vi "BuildWindow.vi"(8 "error in (no error)":errorcluster, 11 "AnalysisPluginsBase in":refnum<class "AnalysisPluginsBase.lvclass">) -> (0 "error out":errorcluster, 3 "AnalysisPluginsBase out":refnum<class "AnalysisPluginsBase.lvclass">)   [LabVIEW 2014]
uses:
  AnalysisPluginsBase.lvclass
  Typedefs/clWindowData.ctl
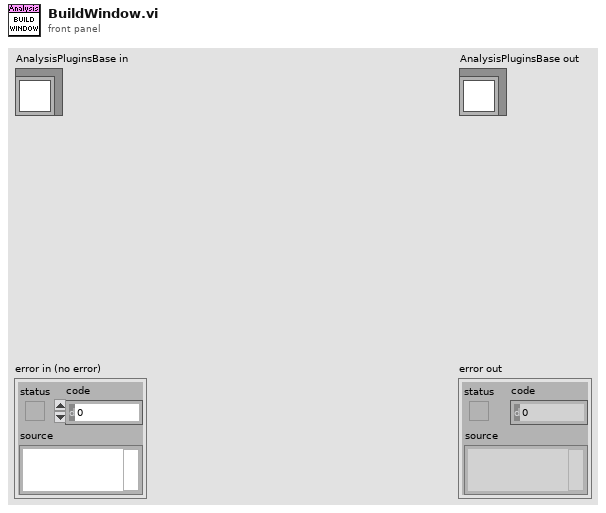
[diagram p1: front panel]
types:
  T1 = typedef "clWindowData.ctl" = cluster{"Timestamp":ext, "Samples":dbl[][], "Window Valid":bool}
  T2 = typedef "AnalysisPlugins.lvlib/AnalysisPluginsBase.lvclass/SampleDataInput.ctl" = T3[]
  T3 = typedef "AnalysisPlugins.lvlib/AnalysisPluginsBase.lvclass/clSampleData.ctl" = cluster{"Timestamp":ext, "SampleDataInput":cluster{"dSampleData":dbl[], "iActualPts":i32}[]}
  T4 = typedef "AnalysisPlugins.lvlib/AnalysisPluginsBase.lvclass/clConfig.ctl" = cluster{"F0":u32, "SettlingTime":dbl, "AnalysisCycles":dbl, "SampleRate":dbl, "NumChannels":u32, "TsOffset":enum16{"start", "middle", "end"}}
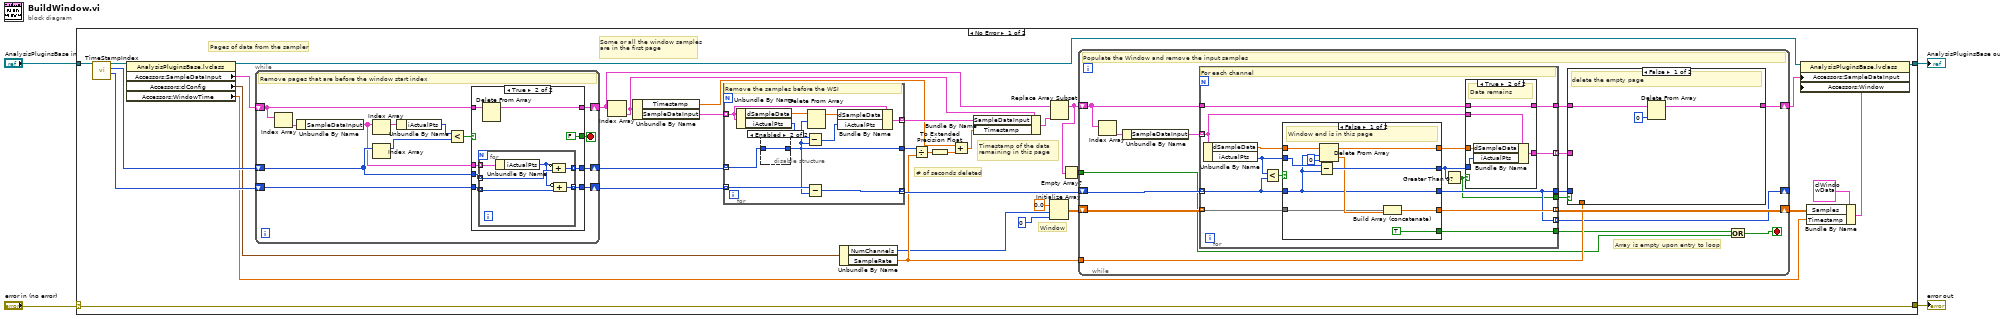
[diagram p0: block diagram]
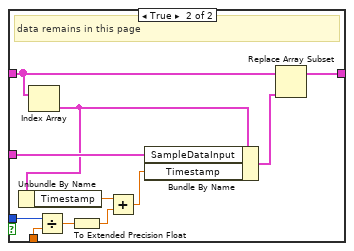
[diagram p2: hidden frame]
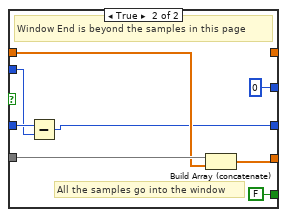
[diagram p4: hidden frame]
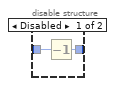
[diagram p5: hidden frame]
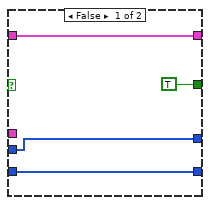
[diagram p6: hidden frame]
diagram:
  n1 = case shown="No Error" "error in (no error)" {
    selector: "error in (no error)" -> [w38 w153]
    tunnel: [w38 w153] -> w3
    tunnel: [w20 w152] -> w1
    tunnel: "AnalysisPluginsBase in" -> [w37 w152]
    frame No Error {
      # "Window"
      # "Timestamp of the data remaining in this page"
      # "# of seconds deleted"
      # "Pages of data from the sampler"
      # "Some or all the window samples are in the first page"
      n2 = call "TimeStampIndex.vi"("Analysis In"=w37) -> ("WEI"=w33:i32[], "WSI"=w34:i32[], "Analysis Out"=w36:refnum<class "AnalysisPluginsBase.lvclass">)  [unwired: 8 in]
      n3 = property class="AnalysisPluginsBase.lvclass"(reference=w36) -> (reference out=w21:refnum<class "AnalysisPluginsBase.lvclass">, "Accessors:SampleDataInput"=w35:T2, "Accessors:clConfig"=w30:T4, "Accessors:WindowTime"=w12:dbl)  [unwired: 1 in, 1 out]
      n4 = while {
        shift-right: [w127] -> w31
        shift-left: w35 -> [w128]
        shift-right: [w121] -> w16
        shift-left: w34 -> [w125]
        shift-right: [w122] -> w32
        shift-left: w33 -> [w123]
        stop <- w126 stop-if-true
        # "Remove pages that are before the window start index"
        n5 = Index Array(array=w128) -> (element=w133:T3)  [unwired: 1 in]
        n6 = Unbundle By Name(w133) -> ("SampleDataInput"=w124:cluster{"dSampleData":dbl[], "iActualPts":i32}[])
        n7 = Index Array(array=w125) -> (element=w130:i32)  [unwired: 1 in]
        n8 = Index Array(array=w124) -> (element=w131:cluster{"dSampleData":dbl[], "iActualPts":i32})  [unwired: 1 in]
        n9 = Unbundle By Name(w131) -> ("iActualPts"=w132:i32)
        n10 = Less?(x=w132, y=w130) -> (x < y?=w129:bool)
        n11 = case shown="True" w129 {
          tunnel: w128 -> [w137 w145]
          tunnel: [w137 w144] -> w127
          tunnel: [TRUE FALSE] -> w126
          tunnel: w125 -> [w136 w142]
          tunnel: w124 -> [_ w141]
          tunnel: w123 -> [w135 w140]
          tunnel: [w135 w139] -> w122
          tunnel: [w136 w138] -> w121
          frame False {
          }
          frame True {
            n12 = for {
              tunnel: w141 -> [w151] mode=indexing
              tunnel: w142 -> [w150] mode=indexing
              tunnel: [w149] -> w138 mode=indexing
              tunnel: w140 -> [w147] mode=indexing
              tunnel: [w146] -> w139 mode=indexing
              n13 = Unbundle By Name(w151) -> ("iActualPts"=w148:i32)
              n14 = Compound Arithmetic op=ADD(invert w148, w150) -> (w149:i32)
              n15 = Compound Arithmetic op=ADD(invert w148, w147) -> (w146:i32)
            }
            n16 = Delete From Array(array=w145) -> (array with subset deleted=w144:T2)  [unwired: 2 in, 1 out]
          }
        }
      }
      n17 = Index Array(array=w31) -> (element=w26:T3)  [unwired: 1 in]
      n18 = Unbundle By Name(w26) -> ("Timestamp"=w15:ext, "SampleDataInput"=w14:cluster{"dSampleData":dbl[], "iActualPts":i32}[])
      n19 = for {
        tunnel: w14 -> [w109] mode=indexing
        tunnel: w16 -> [w116] mode=indexing
        tunnel: w32 -> [w113] mode=indexing
        tunnel: [w114] -> w25 mode=indexing
        tunnel: [w112] -> w22 mode=indexing
        tunnel: [w108] -> w29
        # "Remove the samples before the WSI"
        n20 = Unbundle By Name(w109) -> ("dSampleData"=w117:dbl[], "iActualPts"=w115:i32)
        n21 = disable-structure shown="Enabled" {
          disable-tunnel: w116 -> [w119 w120]
          disable-tunnel: [w118 w120] -> w108
          frame Disabled {
            n22 = Decrement(x=w119) -> (x-1=w118:i32)
          }
          frame Enabled {
          }
        }
        n23 = Subtract(x=w115, y=w108) -> (x-y=w110:i32)
        n24 = Subtract(x=w113, y=w108) -> (x-y=w112:i32)
        n25 = Delete From Array(array=w117, length=w108) -> (array with subset deleted=w111:dbl[])  [unwired: 1 in, 1 out]
        n26 = Bundle By Name(cluster=w109, "dSampleData"=w111, "iActualPts"=w110) -> (w114:cluster{"dSampleData":dbl[], "iActualPts":i32})
      }
      n27 = Unbundle By Name(w30) -> ("NumChannels"=w10:u32, "SampleRate"=w13:dbl)
      n28 = Divide(x=w29, y=w13) -> (x/y=w28:dbl)
      n29 = To Extended Precision Float(1:w28) -> (0:w27:ext)
      n30 = Add(x=w15, y=w27) -> (x+y=w24:ext)
      n31 = Bundle By Name(cluster=w26, "SampleDataInput"=w25, "Timestamp"=w24) -> (w23:T3)
      n32 = Initialize Array(0.0 ("element"), w10, 0 ("dimension size")) -> (w8:dbl[][])
      n33 = Replace Array Subset(array=w31, new element=w23) -> (w6:T2)  [unwired: 1 in]
      n34 = Empty Array?(array=w6) -> (empty?=w5:bool)
      n35 = while {
        shift-right: [w47] -> w19
        shift-left: w6 -> [w51]
        shift-right: [w43] -> _
        shift-left: w22 -> [w52]
        shift-right: [w50] -> w17
        shift-left: w8 -> [w49]
        tunnel: w13 -> [w44]
        tunnel: w5 -> [w39]
        stop <- w40 stop-if-true
        # "Array is empty upon entry to loop"
        # "Populate the Window and remove the input samples"
        n36 = Index Array(array=w51) -> (element=w54:T3)  [unwired: 1 in]
        n37 = Unbundle By Name(w54) -> ("SampleDataInput"=w53:cluster{"dSampleData":dbl[], "iActualPts":i32}[])
        n38 = for {
          tunnel: w53 -> [w74] mode=indexing
          tunnel: w52 -> [w81] mode=indexing
          tunnel: w51 -> [w76]
          tunnel: [w77] -> w41
          tunnel: [w75] -> w48
          tunnel: [w72] -> w46 mode=indexing
          tunnel: [w71] -> w45
          tunnel: [w71] -> w43 mode=indexing
          tunnel: [w69] -> w42
          tunnel: w49 -> [w78] mode=indexing
          tunnel: [w79] -> w50 mode=indexing
          # "For each channel"
          n39 = Unbundle By Name(w74) -> ("dSampleData"=w82:dbl[], "iActualPts"=w80:i32)
          n40 = Less?(x=w80, y=w81) -> (x < y?=w83:bool)
          n41 = case shown="False" w83 {
            tunnel: w82 -> [w99 w103]
            tunnel: w81 -> [w91 w106]
            tunnel: w80 -> [w98 w102]
            tunnel: [w97 _] -> w73
            tunnel: [w96 0] -> w70
            tunnel: [w94 w104] -> w79
            tunnel: w78 -> [w93 w105]
            tunnel: [TRUE FALSE] -> w77
            tunnel: [w91 w101] -> w71
            frame False {
              # "Window end is in this page"
              n42 = Subtract(x=w98, y=w91) -> (x-y=w96:i32)
              n43 = Delete From Array(array=w99, length=w91, index=0) -> (deleted portion=w95:dbl[], array with subset deleted=w97:dbl[])
              n44 = Build Array (concatenate)(w93, w95) -> (w94:dbl[])
            }
            frame True {
              # "All the samples go into the window"
              # "Window End is beyond the samples in this page"
              n45 = Subtract(x=w106, y=w102) -> (x-y=w101:i32)
              n46 = Build Array (concatenate)(w105, w103) -> (w104:dbl[])
            }
          }
          n47 = Greater Than 0?(x=w70) -> (x > 0?=w69:bool)
          n48 = case shown="True" w69 {
            tunnel: w76 -> [w84 w86]
            tunnel: [w84 w86] -> w75
            tunnel: w74 -> [_ w89]
            tunnel: w73 -> [_ w88]
            tunnel: w70 -> [_ w87]
            tunnel: [_ w85] -> w72
            frame False {
              # "Page is empty"
            }
            frame True {
              # "Data remains"
              n49 = Bundle By Name(cluster=w89, "dSampleData"=w88, "iActualPts"=w87) -> (w85:cluster{"dSampleData":dbl[], "iActualPts":i32})
            }
          }
        }
        n50 = case shown="False" w42 {
          tunnel: [w55 w58] -> w47
          tunnel: w48 -> [w56 w60]
          tunnel: w46 -> [_ w68]
          tunnel: w45 -> [_ w66]
          tunnel: w44 -> [_ w65]
          frame False {
            # "delete the empty page"
            n51 = Delete From Array(array=w56, index=0) -> (array with subset deleted=w55:T2)  [unwired: 1 in, 1 out]
          }
          frame True {
            # "data remains in this page"
            n52 = Index Array(array=w60) -> (element=w67:T3)  [unwired: 1 in]
            n53 = Unbundle By Name(w67) -> ("Timestamp"=w63:ext)
            n54 = Divide(x=w66, y=w65) -> (x/y=w64:dbl)
            n55 = To Extended Precision Float(1:w64) -> (0:w62:ext)
            n56 = Add(x=w63, y=w62) -> (x+y=w61:ext)
            n57 = Bundle By Name(cluster=w67, "SampleDataInput"=w68, "Timestamp"=w61) -> (w59:T3)
            n58 = Replace Array Subset(array=w60, new element=w59) -> (w58:T2)  [unwired: 1 in]
          }
        }
        n59 = Or(x=w41, y=w39) -> (x .or. y?=w40:bool)
      }
      n60 = Bundle By Name(cluster=T1 {"Timestamp"=0.0, "Samples"=[], "Window Valid"=FALSE} ("Window"), "Samples"=w17, "Timestamp"=w12) -> (w11:T1)
      n61 = property class="AnalysisPluginsBase.lvclass"(reference=w21, "Accessors:SampleDataInput"=w19, "Accessors:Window"=w11) -> (reference out=w20:refnum<class "AnalysisPluginsBase.lvclass">)  [unwired: 1 in, 1 out]
    }
    frame Error {
    }
  }
  "error out" <- w3
  "AnalysisPluginsBase out" <- w1
